vi "Each_Mergedata_struct_Add.vi"(6 "Active Sensors":bool[](array[boolean]), 7 "Mergedata_struct输入":refnum<k24>[](array[refnum]), 8 "错误输入（无错误）":errorcluster, 9 "Controls[]":refnum<vi>[](array[refnum])) -> (0 "错误输出":errorcluster, 2 "Mergedata_struct输出":refnum<k24>[](array[refnum]))   [LabVIEW 2017]
doc: "for mergedata"
uses:
  D:/test/PDLSTS/LV_PDL LvVer17.0/LV_PDL_x86/DLL/STSProcess.dll
  DLL/STSProcess.dll
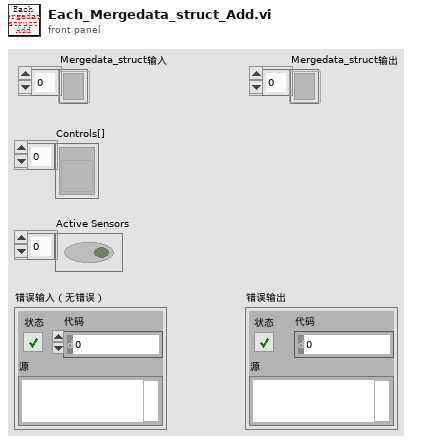
[diagram p1: front panel]
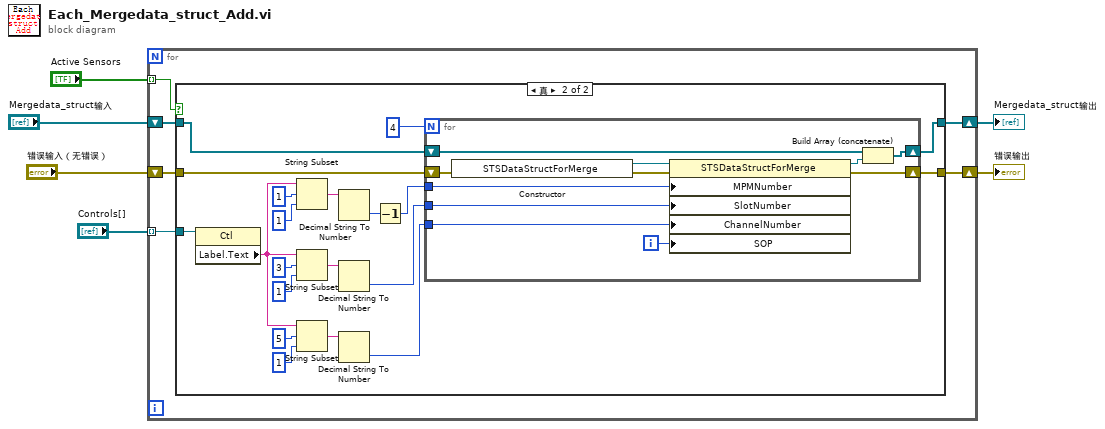
[diagram p0: block diagram]
diagram:
  n1 = for {
    tunnel: "Controls[]" -> [w11] mode=indexing
    tunnel: "Active Sensors" -> [w12] mode=indexing
    shift-right: [w9] -> w4
    shift-left: "Mergedata_struct输入" -> [w10]
    shift-right: [w7] -> w6
    shift-left: "错误输入（无错误）" -> [w8]
    n2 = case shown="真" w12 {
      tunnel: w11 -> [_ w24]
      tunnel: w10 -> [w14 w19]
      tunnel: [w14 w18] -> w9
      tunnel: w8 -> [w13 w17]
      tunnel: [w13 w16] -> w7
      frame False {
      }
      frame True {
        n3 = property class="Ctl"(reference=w24) -> ("Label.Text"=w23:string)  [unwired: 1 in, 2 out]
        n4 = String Subset(string=w23, offset (0)=1 ("偏移量(0)"), length (rest)=1 ("长度（剩余）")) -> (substring=w27:string)
        n5 = String Subset(string=w23, offset (0)=3 ("偏移量(0)"), length (rest)=1 ("长度（剩余）")) -> (substring=w28:string)
        n6 = String Subset(string=w23, offset (0)=5 ("偏移量(0)"), length (rest)=1 ("长度（剩余）")) -> (substring=w26:string)
        n7 = Decimal String To Number(string=w27) -> (number=w25:i32)  [unwired: 2 in, 1 out]
        n8 = Decimal String To Number(string=w28) -> (number=w21:i32)  [unwired: 2 in, 1 out]
        n9 = Decimal String To Number(string=w26) -> (number=w22:i32)  [unwired: 2 in, 1 out]
        n10 = Decrement(x=w25) -> (x-1=w20:i32)
        n11 = for {
          N: 4 -> [_]
          tunnel: w22 -> [w44]
          tunnel: w21 -> [w43]
          tunnel: w20 -> [w42]
          shift-right: [w45] -> w16
          shift-left: w17 -> [w39]
          shift-right: [w40] -> w18
          shift-left: w19 -> [w41]
          i -> [w36]
          n12 = constructor class="STSDataStructForMerge"(error in=w39) -> (reference out=w37:refnum<k24>, error out=w38:errorcluster)  [unwired: 2 in, 1 out]
          n13 = property class="STSDataStructForMerge"(reference=w37, error in=w38, "MPMNumber"=w42, "SlotNumber"=w43, "ChannelNumber"=w44, "SOP"=w36) -> (reference out=w35:refnum<k24>, error out=w45:errorcluster)
          n14 = Build Array (concatenate)(w41, w35) -> (w40:refnum<k24>[])
        }
      }
    }
  }
  "错误输出" <- w6
  "Mergedata_struct输出" <- w4
